vi "Example Threshold.vi"() -> ()   [LabVIEW 2013]
uses:
  C:/tf/play/labview/Tinkerforge.dll
  Tinkerforge.dll
panel:
  in  "stop":bool
  out "callback counter":i32
  out "last voltage (V)":sgl
  in  "uid":string="amb"
  in  "port":i32=4223
  in  "host":string="localhost"
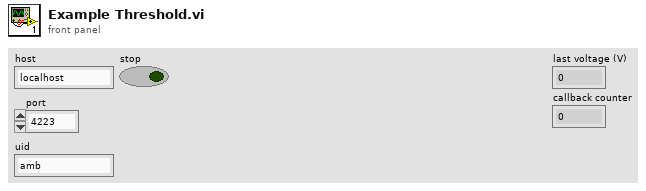
[diagram p1: front panel]
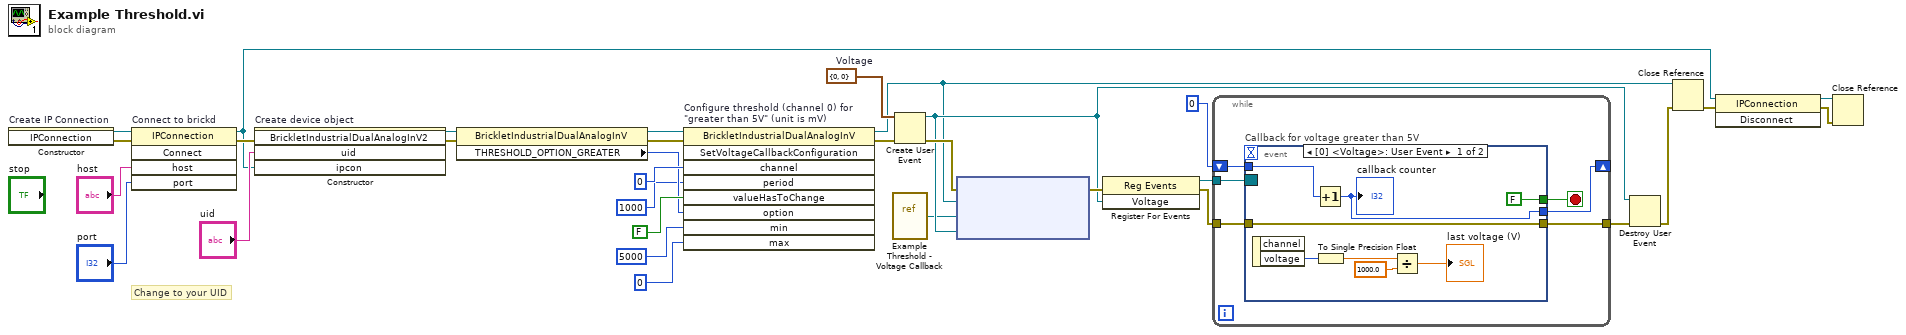
[diagram p0: block diagram]
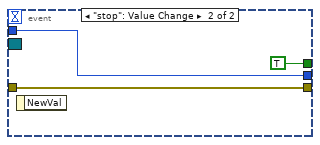
[diagram p2: hidden frame]
diagram:
  w16 = cluster{"channel":u8, "voltage":i32} {"channel"=0, "voltage"=0}  # Voltage
  # "Change to your UID"
  n1 = constructor on="Create IP Connection" class="IPConnection"() -> (reference out=w32:refnum<k24>, error out=w9:errorcluster)  [unwired: 3 in, 1 out]
  n2 = invoke on="Connect to brickd" class="IPConnection" method="Connect"(reference=w32, error in=w9, "host"="host", "port"="port") -> (reference out=w25:refnum<k24>, error out=w28:errorcluster)  [unwired: 1 in, 3 out]
  n3 = constructor on="Create device object" class="BrickletIndustrialDualAnalogInV"(error in=w28, "uid"="uid", "ipcon"=w25) -> (reference out=w6:refnum<k24>, error out=w7:errorcluster)  [unwired: 2 in, 3 out]
  n4 = property class="BrickletIndustrialDualAnalogInV"(reference=w6, error in=w7) -> (reference out=w12:refnum<k24>, error out=w13:errorcluster, "THRESHOLD_OPTION_GREATER"=w2:u16)
  n5 = invoke on="Configure threshold (channel 0) for\n\"greater than 5V\" (unit is mV)" class="BrickletIndustrialDualAnalogInV" method="SetVoltageCallbackConfiguration"(reference=w12, error in=w13, "channel"=u8 0 ("sensor"), "period"=i64 1000, "valueHasToChange"=FALSE, "option"=w2, "min"=5000, "max"=0) -> (reference out=w15:refnum<k24>, error out=w14:errorcluster)  [unwired: 1 in, 7 out]
  n6 = vi-ref "Example Threshold - Voltage Callback.vi"() -> ("vi reference"=w10:refnum<vi>)
  n7 = Create User Event(user event datatype=w16, error in=w14) -> (user event=w18:refnum<user-event>, error out=w23:errorcluster)
  n8 = node ("Register Event Callback")(w23, w15, w10, w18) -> (w22:errorcluster)  [unwired: 1 in, 1 out]
  n9 = register-events(error in=w22, w18) -> (reference out=w21:refnum<event-registration>, error out=w19:errorcluster)  [unwired: 1 in]
  n10 = while {
    tunnel: w21 -> [w38]
    tunnel: [w37] -> w20
    tunnel: w19 -> [w36]
    shift-right: [w34] -> _
    shift-left: 0 -> [w35]
    stop <- w33 stop-if-true
    n11 = event "Callback for voltage greater than 5V" shown="[0] <Voltage>: User Event" {
      selector: w38 -> [_ _]
      dyn-events: _ -> [_ _]
      timeout: _ -> [_ _]
      tunnel: [w43 w48] -> w37
      tunnel: w36 -> [w43 w48]
      tunnel: w35 -> [w41 w47]
      tunnel: [w40 w47] -> w34
      tunnel: [FALSE TRUE] -> w33
      event User Event {
        n12 = event-data() -> ("voltage"=w44:i32)  [unwired: 1 in, 1 out]
        n13 = Increment(x=w41) -> (x+1=w40:i32)
        "callback counter" <- w40
        n14 = To Single Precision Float(number=w44) -> (single precision float=w45:sgl)
        n15 = Divide(x=w45, y=sgl 1000.0) -> (x/y=→"last voltage (V)":sgl)
      }
      event "stop": Value Change {
        n16 = event-data() -> ()  [unwired: 1 in, 1 out]
      }
    }
  }
  n17 = Destroy User Event(user event=w18, error in=w20) -> (error out=w17:errorcluster)
  n18 = Close Reference(reference=w15, error in (no error)=w17) -> (error out=w27:errorcluster)
  n19 = invoke class="IPConnection" method="Disconnect"(reference=w25, error in=w27) -> (reference out=w24:refnum<k24>, error out=w26:errorcluster)  [unwired: 1 in, 1 out]
  n20 = Close Reference(reference=w24, error in (no error)=w26) -> ()  [unwired: 1 out]
